vi "XNET TCP Socket Write.vi"   [LabVIEW 2018]
doc: "Writes data to a TCP network connection."
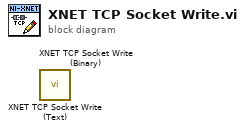
[diagram p0: block diagram]
diagram:
  n1 = call "XNET TCP Socket Write (Text).vi"() -> ()  [unwired: 9 in, 3 out]
  n2 = call "XNET TCP Socket Write (Binary).vi"() -> ()  [unwired: 9 in, 3 out]
